vi "Kernel.vi"(0 "reference in":refnum<class "G#Object.lvclass">, 1 "object name":string, 2 "option 1":bool, 3 "option 2":bool, 4 "depth":i32, 5 "error in (no error)":errorcluster, 6 "state":T2, 7 "option 3":bool, 8 "attributes in":variant[](array[variant]), 10 "class attributes in":variant[](array[variant])) -> (11 "class attributes out":variant[](array[variant]), 12 "class hierarchy":T1[](array[typedef]), 13 "attributes out":variant[](array[variant]), 14 "reference out":refnum<class "G#Object.lvclass">, 15 "attribute refs":u32[](array[numeric]), 16 "static attribute ref":u32, 17 "output 1":bool, 18 "output 2":bool, 19 "error out":errorcluster)   [LabVIEW 2020, in "G#Object.lvclass"]
doc: "This is the G#object kernel that is responsible for creating and deleting object."
uses:
  <vilib>/addons/_AddQ/G#Object/G#Object.lvclass
  <vilib>/addons/_AddQ/G#Object/utils/G#Object_State.ctl
  <vilib>/addons/_AddQ/G#Object/utils/G#Object_ClassHierarchy.ctl
  <vilib>/addons/_AddQ/G#Object/G#Object.lvclass/G#Object.ctl
  <vilib>/addons/_AddQ/G#Object/utils/G#Object_ObjectInfoType.ctl
  <vilib>/addons/_AddQ/G#Object/utils/G#Object_CreateMethod.ctl
  <vilib>/addons/_AddQ/G#Object/utils/G#Object_EventType.ctl
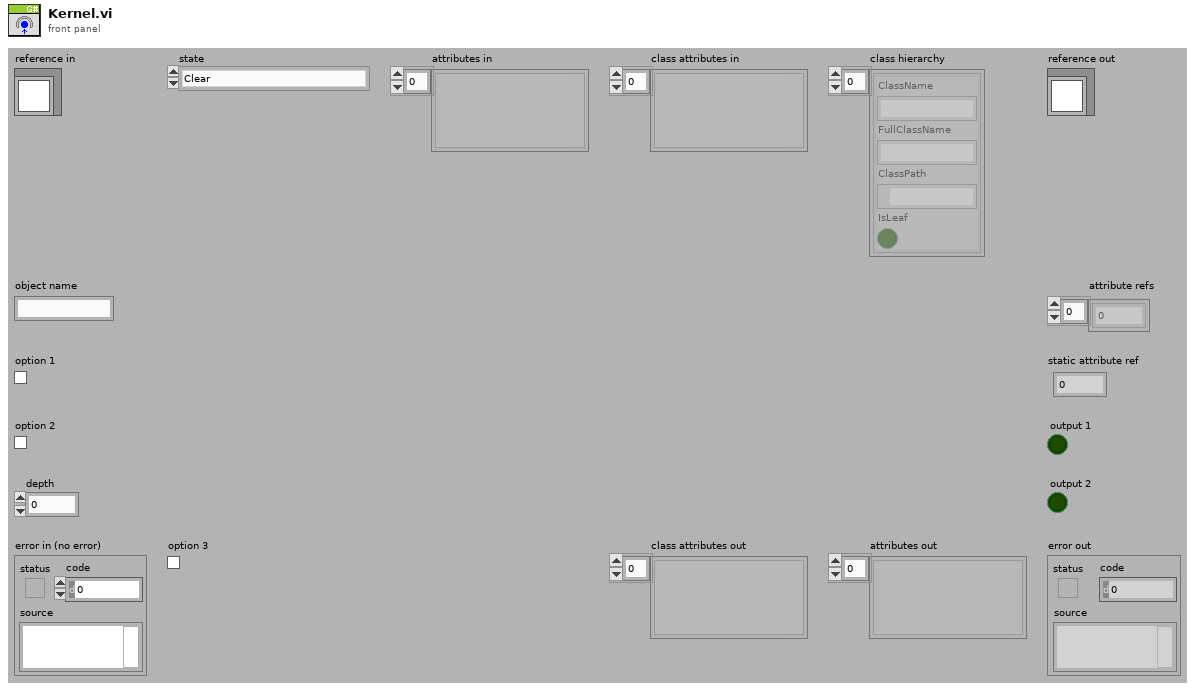
[diagram p1: front panel]
types:
  T1 = typedef "G#Object.lvclass/G#Object_ClassHierarchy.ctl" = cluster{"ClassName":string, "FullClassName":string, "ClassPath":path, "IsLeaf":bool}
  T2 = typedef "G#Object.lvclass/G#Object_State.ctl" = enum16{"Clear", "Create", "Delete", "Get class attributes", "Class hierarchy", "Get attribute value", "Set attribute value"}
  T3 = typedef "G#Object.lvclass/G#Object_ObjectInfoType.ctl" = cluster{"ObjectName":string, "ObjectID":u32, "Users":i32, "Counter":bool, "AttributeRefs":u32[], "FullClassName":string, "ClassName":string, "CreateMethod":T4, "GenericDestructorExists":bool, "Owner":string}
  T4 = typedef "G#Object.lvclass/G#Object_CreateMethod.ctl" = enum16{"Create", "Create or look up existing", "Look up existing"}
  T5 = typedef "G#Object.lvclass/G#Object_EventType.ctl" = enum16{"Created new", "Looked up existing", "Deleted", "Forced delete", "Not deleted", "Garbage collected", "Cleared", "User", "Error", "External create object", "External create class attributes", "Created class attributes", "Run constructor", "Run constructor done", "Run open method", "Run open method done"}
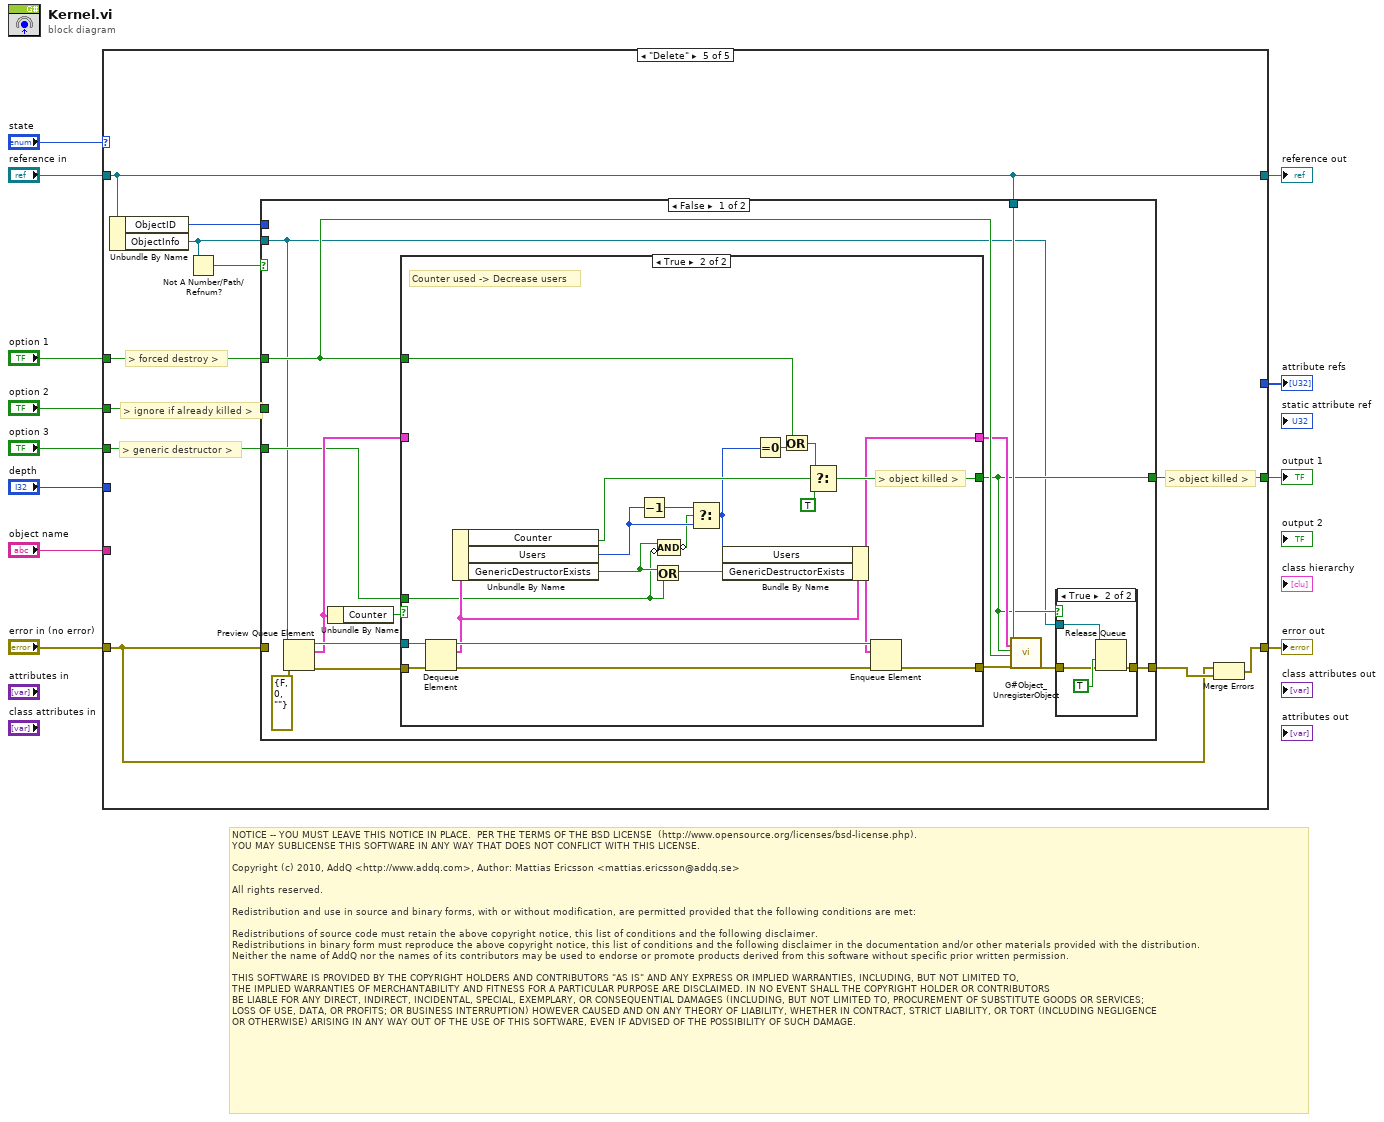
[diagram p0: block diagram]
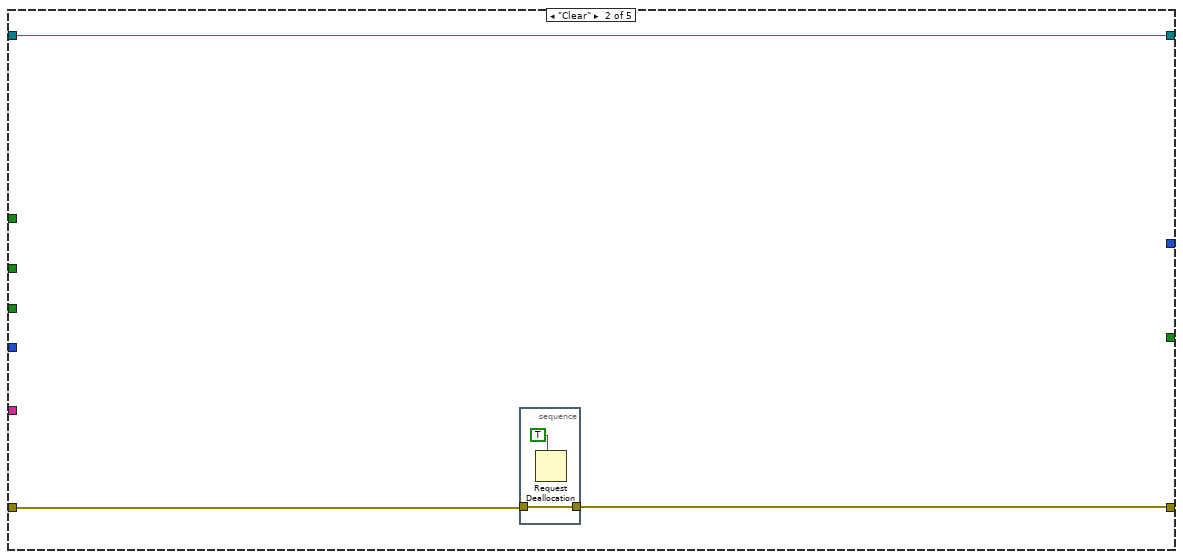
[diagram p3: hidden frame]
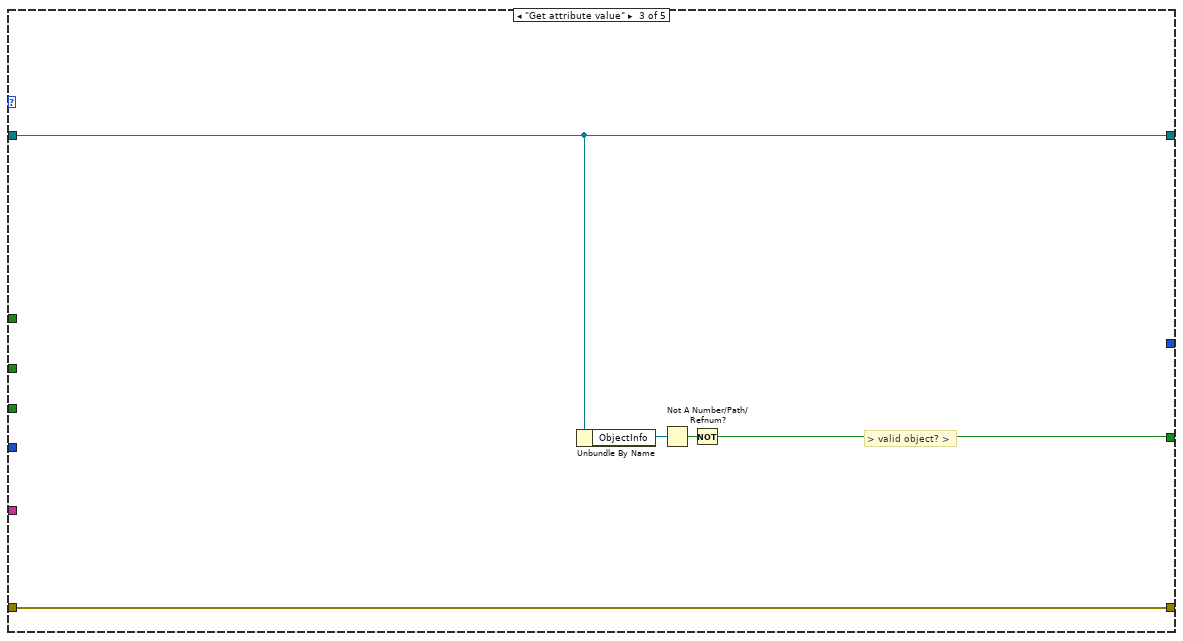
[diagram p4: hidden frame]
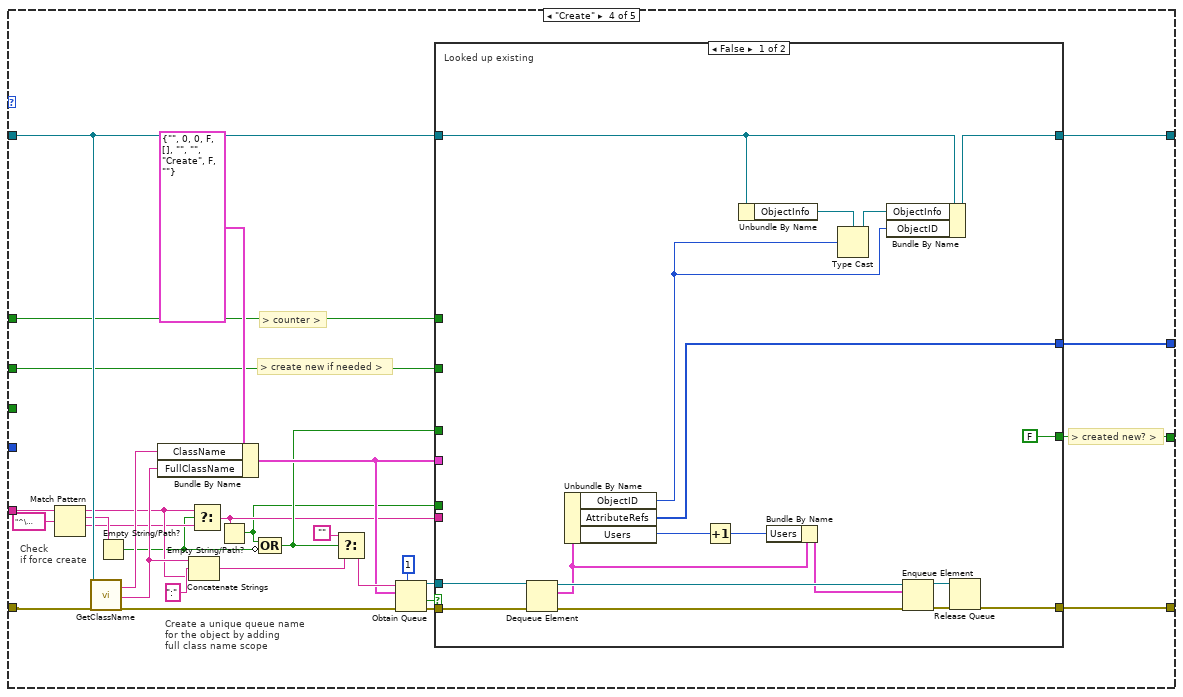
[diagram p5: hidden frame]
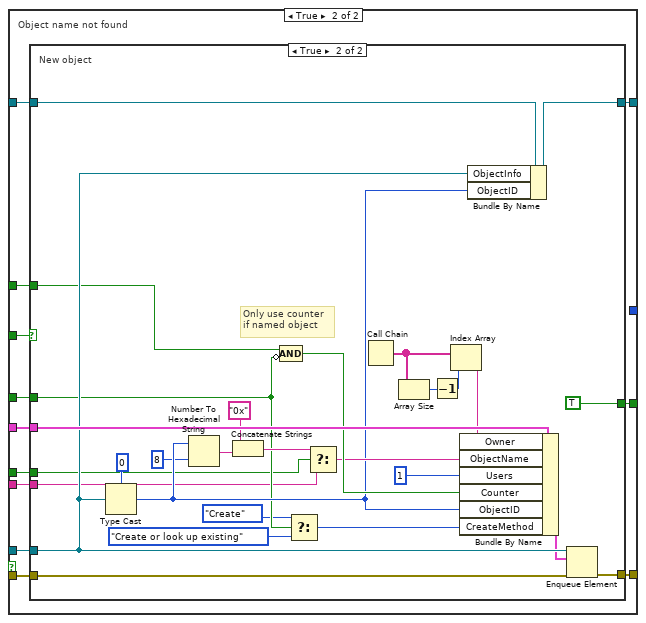
[diagram p6: hidden frame]
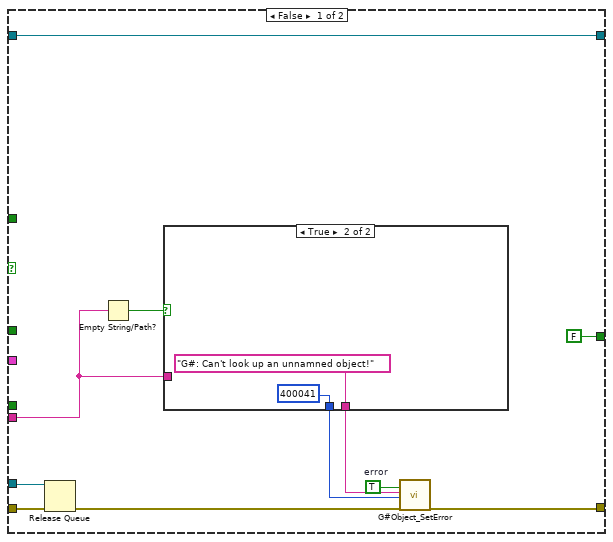
[diagram p7: hidden frame]
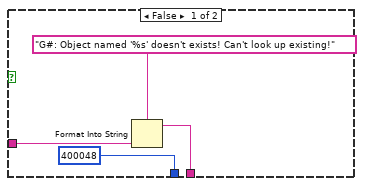
[diagram p8: hidden frame]
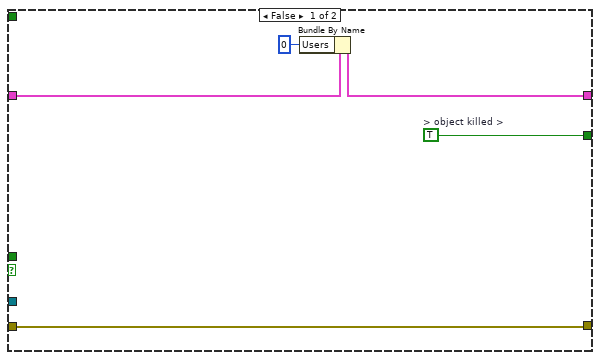
[diagram p10: hidden frame]
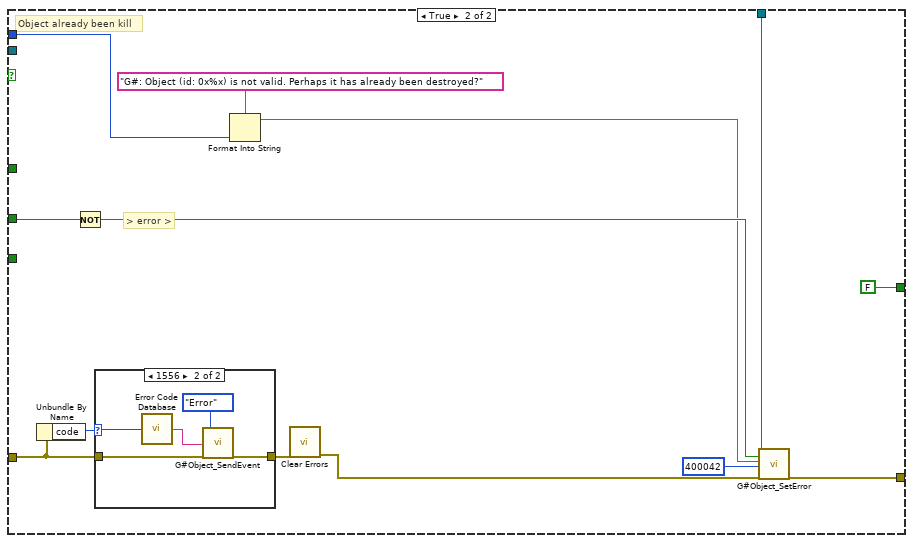
[diagram p11: hidden frame]
diagram:
  # "NOTICE -- YOU MUST LEAVE THIS NOTICE IN PLACE.  PER THE TERMS OF THE BSD LICENSE  (http://www.opensource.org/licenses/bsd-license.php).\nYOU MAY SUBLICENSE THIS SOFTWARE IN ANY WAY THAT DOES NOT CONFLICT WITH THIS LICENSE.\n\nCopyright (c) 2010, AddQ <http://www.addq.com>, Author: Mattias Ericsson <mattias.ericsson@addq.se>\n\nAll rights reserved.\n\nRedistribution and use in source and binary forms, with or without modification, are permitted provided that the following conditions are met:\n\nRedistributions of source code must retain the above copyright notice, this list of conditions and the following disclaimer.\nRedistributions in binary form must reproduce the above copyright notice, this list of conditions and the following disclaimer in the documentation and/or other materials provided with the distribution.\nNeither the name of AddQ nor the names of its contributors may be used to endorse or promote products derived from this software without specific prior written permission.\n \nTHIS SOFTWARE IS PROVIDED BY THE COPYRIGHT HOLDERS AND CONTRIBUTORS \"AS IS\" AND ANY EXPRESS OR IMPLIED WARRANTIES, INCLUDING, BUT NOT LIMITED TO,\nTHE IMPLIED WARRANTIES OF MERCHANTABILITY AND FITNESS FOR A PARTICULAR PURPOSE ARE DISCLAIMED. IN NO EVENT SHALL THE COPYRIGHT HOLDER OR CONTRIBUTORS\nBE LIABLE FOR ANY DIRECT, INDIRECT, INCIDENTAL, SPECIAL, EXEMPLARY, OR CONSEQUENTIAL DAMAGES (INCLUDING, BUT NOT LIMITED TO, PROCUREMENT OF SUBSTITUTE GOODS OR SERVICES;\nLOSS OF USE, DATA, OR PROFITS; OR BUSINESS INTERRUPTION) HOWEVER CAUSED AND ON ANY THEORY OF LIABILITY, WHETHER IN CONTRACT, STRICT LIABILITY, OR TORT (INCLUDING NEGLIGENCE\nOR OTHERWISE) ARISING IN ANY WAY OUT OF THE USE OF THIS SOFTWARE, EVEN IF ADVISED OF THE POSSIBILITY OF SUCH DAMAGE."
  n1 = case shown="\"Delete\"" "state" {
    tunnel: "reference in" -> [w14 w17 w23 w40 w136]
    tunnel: [w14 w17 w23 w41 w136] -> w10
    tunnel: "error in (no error)" -> [w13 w16 w24 w45 w130]
    tunnel: [w13 w15 w24 w44 w139] -> w11
    tunnel: [_ _ w20 w36 w137] -> w8
    tunnel: [_ _ _ w42 _] -> w7
    tunnel: "option 1" -> [_ _ _ w39 w138]
    tunnel: "option 2" -> [_ _ _ w37 w134]
    tunnel: "object name" -> [_ _ _ w35 _]
    tunnel: "depth" -> [_ _ _ _ _]
    tunnel: "option 3" -> [_ _ _ _ w131]
    frame Default {
    }
    frame "Clear" {
      n2 = stacked-sequence {
        tunnel: w16 -> [w18]
        tunnel: [w18] -> w15
        frame #0 {
          n3 = Request Deallocation(TRUE ("flag")) -> ()
        }
      }
    }
    frame "Get attribute value" {
      # "> valid object? >"
      n4 = Unbundle By Name(w23) -> ("ObjectInfo"=w22:refnum<queue>)
      n5 = Not A Number/Path/Refnum?(number/path/refnum=w22) -> (NaN/Path/Refnum?=w21:bool)
      n6 = Not(x=w21) -> (.not. x?=w20:bool)
    }
    frame "Create" {
      # "Check\nif force create"
      # "> created new? >"
      # "> create new if needed >"
      # "> counter >"
      # "Create a unique queue name\nfor the object by adding\nfull class name scope"
      n7 = Match Pattern(string=w35, regular expression="^\u0000") -> (before substring=w30:string, match substring=w33:string, after substring=w29:string)  [unwired: 1 in, 1 out]
      n8 = call-dynamic "GetClassName.vi"("reference in"=w40, "error in (no error)"=w45) -> ("class name"=w46:string, "full class name"=w38:string, "error out"=w50:errorcluster)  [unwired: 13 in, 2 out]
      n9 = Empty String/Path?(string/path=w33) -> (empty?=w28:bool)
      n10 = Bundle By Name(cluster=T3 {"ObjectName"="", "ObjectID"=0, "Users"=0, "Counter"=FALSE, "AttributeRefs"=[], "FullClassName"="", "ClassName"="", "CreateMethod"=enum."Create", "GenericDestructorExists"=FALSE, "Owner"=""}, "ClassName"=w46, "FullClassName"=w38) -> (w47:T3)
      n11 = Concatenate Strings(w38, ":", w30) -> (w31:string)
      n12 = Select(t=w30, s=w28, f=w29) -> (s? t:f=w26:string)
      n13 = Empty String/Path?(string/path=w26) -> (empty?=w25:bool)
      n14 = Compound Arithmetic op=OR(w25, invert w28) -> (w27:bool)
      n15 = Select(t="", s=w27, f=w31) -> (s? t:f=w48:string)
      n16 = Obtain Queue(max queue size (-1, unlimited)=1, name (unnamed)=w48, element data type=w47, error in (no error)=w50) -> (queue out=w51:refnum<queue>, created new?=w43:bool, error out=w52:errorcluster)  [unwired: 1 in]
      n17 = case shown="False" w43 {
        tunnel: [w65 w84] -> w44
        tunnel: w52 -> [w72 w83]
        tunnel: w51 -> [w71 w79]
        tunnel: w47 -> [_ w82]
        tunnel: w40 -> [w62 w81]
        tunnel: [w61 w80] -> w41
        tunnel: [w59 _] -> w42
        tunnel: w39 -> [_ w78]
        tunnel: w27 -> [_ w77]
        tunnel: w26 -> [_ w76]
        tunnel: w37 -> [_ w75]
        tunnel: [FALSE w74] -> w36
        tunnel: w25 -> [_ w73]
        frame False {
          # "Looked up existing"
          n18 = Dequeue Element(queue=w71, error in (no error)=w72) -> (queue out=w69:refnum<queue>, element=w68:T3, error out=w70:errorcluster)  [unwired: 1 in, 1 out]
          n19 = Unbundle By Name(w68) -> ("ObjectID"=w57:u32, "AttributeRefs"=w59:u32[], "Users"=w67:i32)
          n20 = Increment(x=w67) -> (x+1=w55:i32)
          n21 = Unbundle By Name(w62) -> ("ObjectInfo"=w63:refnum<queue>)
          n22 = Bundle By Name(cluster=w68, "Users"=w55) -> (w58:T3)
          n23 = Type Cast(type=w63, x=w57) -> (*(type *) &x=w60:refnum<queue>)
          n24 = Bundle By Name(cluster=w62, "ObjectInfo"=w60, "ObjectID"=w57) -> (w61:refnum<class "G#Object.lvclass">)
          n25 = Enqueue Element(queue=w69, element=w58, error in (no error)=w70) -> (queue out=w64:refnum<queue>, error out=w66:errorcluster)  [unwired: 1 in, 1 out]
          n26 = Release Queue(queue=w64, error in (no error)=w66) -> (error out=w65:errorcluster)  [unwired: 1 in, 2 out]
        }
        frame True {
          # "Object name not found"
          n27 = case shown="True" w75 {
            tunnel: [w94 w129] -> w84
            tunnel: w83 -> [w88 w128]
            tunnel: w82 -> [_ w126]
            tunnel: w81 -> [w92 w124]
            tunnel: [w92 w123] -> w80
            tunnel: w79 -> [w86 w122]
            tunnel: w78 -> [_ w119]
            tunnel: w77 -> [_ w112]
            tunnel: w76 -> [w90 w103]
            tunnel: [FALSE TRUE] -> w74
            tunnel: w73 -> [_ w102]
            frame False {
              w93 = TRUE  # error
              n28 = Release Queue(queue=w86, error in (no error)=w88) -> (error out=w87:errorcluster)  [unwired: 1 in, 2 out]
              n29 = Empty String/Path?(string/path=w90) -> (empty?=w89:bool)
              n30 = case shown="True" w89 {
                tunnel: [w98 "G#: Can't look up an unnamned object!"] -> w91
                tunnel: w90 -> [w97 _]
                tunnel: [400048 ("code") 400041 ("code")] -> w85
                frame False {
                  n31 = Format Into String(format string="G#: Object named '%s' doesn't exists! Can't look up existing!", w97) -> (resulting string=w98:string)  [unwired: 2 in, 1 out]
                }
                frame True {
                }
              }
              n32 = call <vilib>:"G#Object_SetError.vi"("error (F)"=w93, "source"=w91, "code"=w85, "error in (no error)"=w87) -> ("error out"=w94:errorcluster)  [unwired: 15 in]
            }
            frame True {
              # "Only use counter\nif named object"
              # "New object"
              n33 = Type Cast(type=u32 0, x=w122) -> (*(type *) &x=w113:u32)
              n34 = Number To Hexadecimal String(1:i16 8 ("width (-)"), 2:w113) -> (0:w117:string)
              n35 = Concatenate Strings("0x" ("string"), w117) -> (w116:string)
              n36 = Compound Arithmetic op=AND(w119, invert w112) -> (w120:bool)
              n37 = Select(t=G#Object_CreateMethod."Create" ("CreateMethod"), s=w112, f=G#Object_CreateMethod."Create or look up existing" ("CreateMethod")) -> (s? t:f=w111:T4)
              n38 = Select(t=w116, s=w102, f=w103) -> (s? t:f=w118:string)
              n39 = Call Chain() -> (call chain=w106:string[])
              n40 = Array Size(array=w106) -> (size(s)=w105:i32)
              n41 = Decrement(x=w105) -> (x-1=w104:i32)
              n42 = Index Array(array=w106, index=w104) -> (element=w107:string)
              n43 = Bundle By Name(cluster=w126, "Owner"=w107, "ObjectName"=w118, "Users"=1, "Counter"=w120, "ObjectID"=w113, "CreateMethod"=w111) -> (w121:T3)
              n44 = Bundle By Name(cluster=w124, "ObjectInfo"=w122, "ObjectID"=w113) -> (w123:refnum<class "G#Object.lvclass">)
              n45 = Enqueue Element(queue=w122, element=w121, error in (no error)=w128) -> (error out=w129:errorcluster)  [unwired: 1 in, 2 out]
            }
          }
        }
      }
    }
    frame "Delete" {
      # "> generic destructor >"
      # "> ignore if already killed >"
      # "> object killed >"
      # "> forced destroy >"
      n46 = Unbundle By Name(w136) -> ("ObjectID"=w133:u32, "ObjectInfo"=w135:refnum<queue>)
      n47 = Not A Number/Path/Refnum?(number/path/refnum=w135) -> (NaN/Path/Refnum?=w132:bool)
      n48 = case shown="False" w132 {
        tunnel: w135 -> [w141 _]
        tunnel: [w143 w196] -> w140
        tunnel: w138 -> [w149 _]
        tunnel: [w142 FALSE ("f")] -> w137
        tunnel: w136 -> [w148 w190]
        tunnel: w134 -> [_ w195]
        tunnel: w133 -> [_ w194]
        tunnel: w131 -> [w145 _]
        tunnel: w130 -> [_ w188]
        frame False {
          n49 = Preview Queue Element(queue=w141, error in (no error)=errorcluster {"status"=FALSE, "code"=0, "source"=""}) -> (queue out=w152:refnum<queue>, element=w151:T3, error out=w153:errorcluster)  [unwired: 1 in, 1 out]
          n50 = Unbundle By Name(w151) -> ("Counter"=w154:bool)
          n51 = case shown="True" w154 {
            tunnel: [w160 w165] -> w147
            tunnel: w153 -> [w160 w175]
            tunnel: w152 -> [_ w176]
            tunnel: w149 -> [_ w180]
            tunnel: [w164 w178] -> w142
            tunnel: [w162 w173] -> w146
            tunnel: w151 -> [w163 _]
            tunnel: w145 -> [_ w167]
            frame False {
              w164 = TRUE  # > object killed >
              n52 = Bundle By Name(cluster=w163, "Users"=0) -> (w162:T3)
            }
            frame True {
              # "> object killed >"
              # "Counter used -> Decrease users"
              n53 = Dequeue Element(queue=w176, error in (no error)=w175) -> (queue out=w183:refnum<queue>, element=w174:T3, error out=w184:errorcluster)  [unwired: 1 in, 1 out]
              n54 = Unbundle By Name(w174) -> ("Counter"=w177:bool, "Users"=w169:i32, "GenericDestructorExists"=w168:bool)
              n55 = Decrement(x=w169) -> (x-1=w171:i32)
              n56 = Or(x=w168, y=w167) -> (x .or. y?=w172:bool)
              n57 = Compound Arithmetic op=AND(w168, invert w167) -> (invert w166:bool)
              n58 = Select(t=w171, s=w166, f=w169) -> (s? t:f=w170:i32)
              n59 = Bundle By Name(cluster=w174, "Users"=w170, "GenericDestructorExists"=w172) -> (w173:T3)
              n60 = Equal To 0?(x=w170) -> (x = 0?=w181:bool)
              n61 = Or(x=w180, y=w181) -> (x .or. y?=w179:bool)
              n62 = Select(t=w179, s=w177, f=TRUE) -> (s? t:f=w178:bool)
              n63 = Enqueue Element(queue=w183, element=w173, error in (no error)=w184) -> (error out=w165:errorcluster)  [unwired: 1 in, 2 out]
            }
          }
          n64 = call <vilib>:"G#Object_UnregisterObject.vi"("reference in"=w148, "object information"=w146, "object killed"=w142, "forced destroy"=w149, "error in (no error)"=w147) -> ("error out"=w144:errorcluster)  [unwired: 13 in, 1 out]
          n65 = case shown="True" w142 {
            tunnel: w144 -> [w155 w158]
            tunnel: [w155 w157] -> w143
            tunnel: w141 -> [_ w156]
            frame False {
            }
            frame True {
              n66 = Release Queue(queue=w156, force destroy? (F)=TRUE, error in (no error)=w158) -> (error out=w157:errorcluster)  [unwired: 2 out]
            }
          }
        }
        frame True {
          # "> error >"
          # "Object already been kill"
          n67 = Unbundle By Name(w188) -> ("code"=w189:i32)
          n68 = Not(x=w195) -> (.not. x?=w193:bool)
          n69 = case shown="1556" w189 {
            selector: w189 -> [_ w200]
            tunnel: w188 -> [w198 w201]
            tunnel: [w198 w199] -> w187
            frame 0, Default {
            }
            frame 1556 {
              n70 = call <vilib>:"Error Code Database.vi"("Error Code"=w200) -> ("Error Text"=w202:string)
              n71 = call <vilib>:"G#Object_SendEvent.vi"("comment"=w202, "error in (no error)"=w201, "G# event type"=G#Object_EventType."Error") -> ("error out"=w199:errorcluster)  [unwired: 16 in]
            }
          }
          n72 = Format Into String(format string="G#: Object (id: 0x%x) is not valid. Perhaps it has already been destroyed?" ("source"), w194) -> (resulting string=w191:string)  [unwired: 2 in, 1 out]
          n73 = call <vilib>:"Clear Errors.vi"("error in (no error)"=w187) -> ("error out"=w186:errorcluster)  [unwired: 5 in, 1 out]
          n74 = call <vilib>:"G#Object_SetError.vi"("reference in"=w190, "error (F)"=w193, "source"=w191, "code"=400042, "error in (no error)"=w186) -> ("error out"=w196:errorcluster)  [unwired: 14 in]
        }
      }
      n75 = Merge Errors(w130, w140) -> (w139:errorcluster)
    }
  }
  "error out" <- w11
  "reference out" <- w10
  "attribute refs" <- w7
  "output 1" <- w8
